vi "Get Nested Object Queue.vi"(8 "error in (no error)":errorcluster, 9 "Name":string, 11 "Measure Object in":refnum<class "Measure Object.lvclass">) -> (0 "error out":errorcluster, 1 "Object Enqueuer":refnum<class "Message Enqueuer.lvclass">, 2 "Found?":bool, 3 "Measure Object out":refnum<class "Measure Object.lvclass">)   [LabVIEW 2016, in "Measure Object.lvclass"]
uses:
  Measure Object.lvclass
  D:/Program Files/National Instruments/LabVIEW 2016/vi.lib/ActorFramework/Actor/Actor.lvclass
  <vilib>/ActorFramework/Message Enqueuer/Message Enqueuer.lvclass
  Measure Object.lvclass/Measure Object.ctl
  <vilib>/ActorFramework/Actor/Actor.lvclass/Actor.ctl
  <vilib>/ActorFramework/Message Enqueuer/Message Enqueuer.lvclass/Message Enqueuer.ctl
  Read Name.vi
  <vilib>/ActorFramework/Message Enqueuer/Init from Existing Queue.vi
  <vilib>/ActorFramework/Actor/Actor.lvclass
panel:
  in  "Self Enqueuer":refnum<class "Message Enqueuer.lvclass">
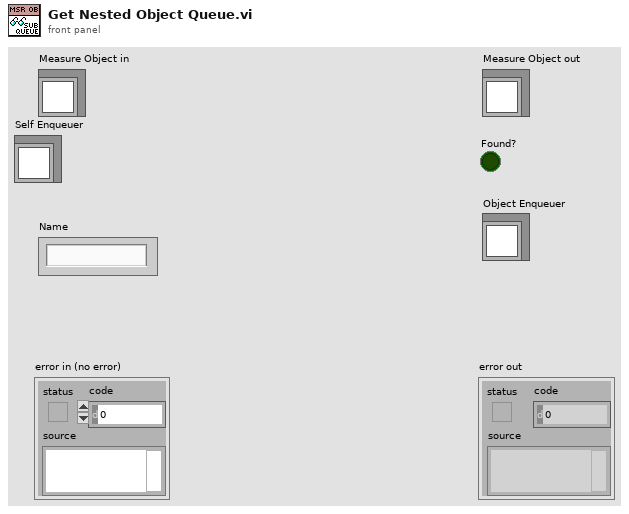
[diagram p1: front panel]
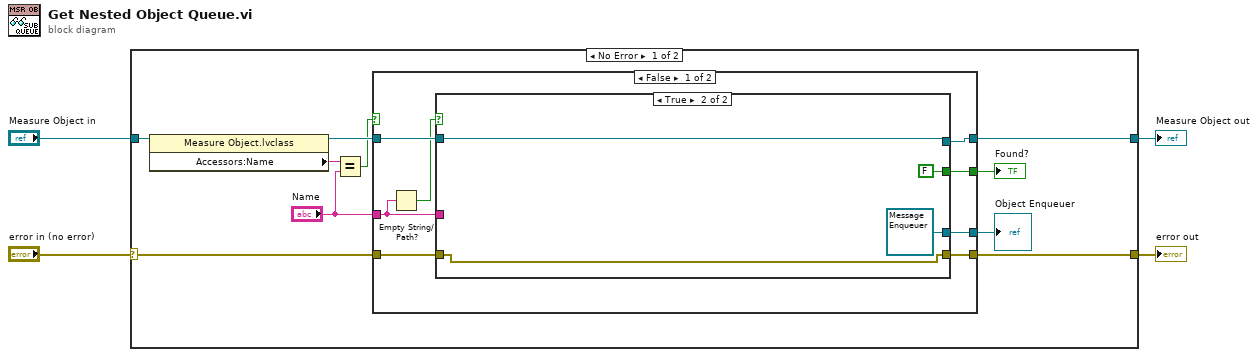
[diagram p0: block diagram]
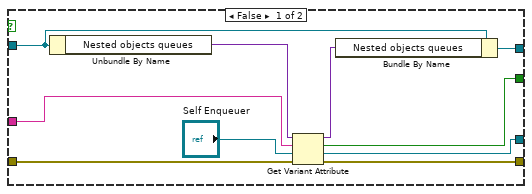
[diagram p2: hidden frame]
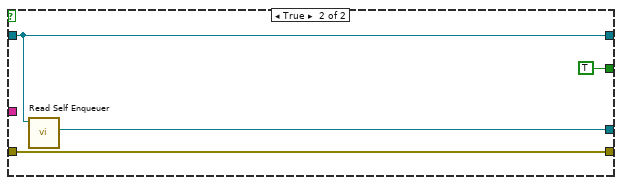
[diagram p3: hidden frame]
diagram:
  n1 = case shown="No Error" "error in (no error)" {
    selector: "error in (no error)" -> [w14 w42]
    tunnel: [w12 w42] -> w3
    tunnel: [w13 w41] -> w1
    tunnel: "Measure Object in" -> [w11 w41]
    frame No Error {
      n2 = property class="Measure Object.lvclass"(reference=w11) -> (reference out=w10:refnum<class "Measure Object.lvclass">, "Accessors:Name"=w9:string)  [unwired: 1 in, 1 out]
      n3 = Equal?(x=w9, y="Name") -> (x = y?=w5:bool)
      n4 = case shown="False" w5 {
        tunnel: w14 -> [w22 w37]
        tunnel: [w21 w38] -> w13
        tunnel: [w20 w37] -> w12
        tunnel: w10 -> [w19 w38]
        tunnel: "Name" -> [w16 _]
        tunnel: [w18 TRUE] -> w7
        tunnel: [w17 w40] -> w6
        frame False {
          n5 = Empty String/Path?(string/path=w16) -> (empty?=w15:bool)
          n6 = case shown="True" w15 {
            tunnel: w22 -> [w31 w33]
            tunnel: [w30 w36] -> w21
            tunnel: [w28 w33] -> w20
            tunnel: w19 -> [w27 w36]
            tunnel: w16 -> [w26 _]
            tunnel: [w24 FALSE] -> w18
            tunnel: [w23 refnum<class "Message Enqueuer.lvclass"> refnum ("Self Enqueuer")] -> w17
            frame False {
              n7 = Unbundle By Name(w27) -> ("Nested objects queues"=w32:variant)
              n8 = Get Variant Attribute(Variant=w32, name=w26, default value (empty Variant)="Self Enqueuer", error in=w31) -> (duplicate Variant=w29:variant, found=w24:bool, value=w23:refnum<class "Message Enqueuer.lvclass">, error out=w28:errorcluster)
              n9 = Bundle By Name(cluster=w27, "Nested objects queues"=w29) -> (w30:refnum<class "Measure Object.lvclass">)
            }
            frame True {
            }
          }
        }
        frame True {
          n10 = call <vilib>:"Read Self Enqueuer.vi"("Actor"=w38) -> ("Self Enqueuer"=w40:refnum<class "Message Enqueuer.lvclass">)  [unwired: 10 in]
        }
      }
      "Found?" <- w7
      "Object Enqueuer" <- w6
    }
    frame Error {
    }
  }
  "error out" <- w3
  "Measure Object out" <- w1
